vi "DTV&EnQueue.vi"(0 "ModuleAdmin In":refnum<class "ModuleAdmin.lvclass">, 1 "Enqueue Type (Enqueue)":T1=enum."Enqueue", 5 "Message":string, 7 "Message Data":variant, 9 "Class":refnum<class "SensorBase.lvclass">, 11 "Error In":errorcluster, 12 "QueueArrayEntry(QMH)":T2) -> (4 "ModuleAdmin Out":refnum<class "ModuleAdmin.lvclass">, 6 "MessageQueue Out":refnum<queue>, 8 "VariantData":variant, 15 "Error Out":errorcluster)   [LabVIEW 2018, in "SensorPlugins.lvlib"]
doc: "Converts the module data to a variant and places the data in a queue based upon the queue entry and the Enqueue type."
uses:
  SensorPlugins.lvlib
  SensorBaseClass/SensorBase.lvclass
  <userlib>/NIST/ModuleAdminLib/ModuleAdmin/ModuleAdmin.lvclass
  <userlib>/NIST/ModuleAdminLib/ModuleAdmin/TypeDefinitions/QueueEntry.ctl
  <userlib>/NIST/ModuleAdminLib/ModuleAdmin/TypeDefinitions/QueueType.ctl
  clMessage.ctl
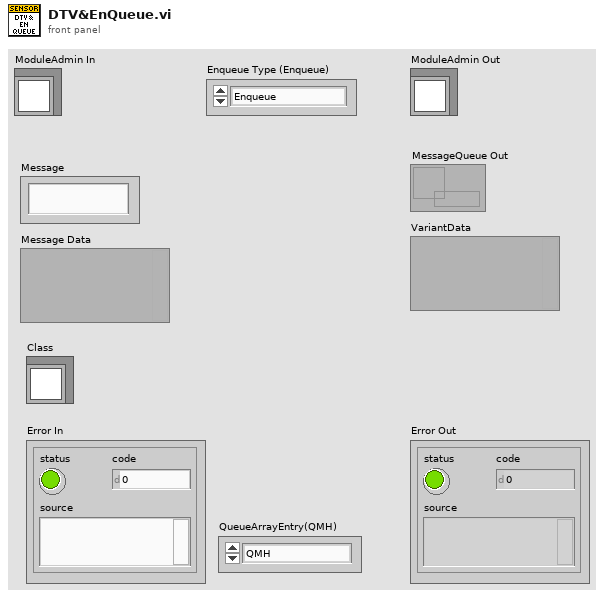
[diagram p1: front panel]
types:
  T1 = typedef "ModuleAdmin.lvlib/ModuleAdmin.lvclass/QueueType.ctl" = enum16{"EnqueueAtFront", "Enqueue", "Lossy Enqueue"}
  T2 = typedef "ModuleAdmin.lvlib/ModuleAdmin.lvclass/QueueEntry.ctl" = enum16{"QMH", "Class Data", "Data Loop", "Queue 4", "Queue 5", "Queue 6", "Queue 7", "Queue 8", "Queue 9", "Queue 10"}
  T3 = typedef "SensorPlugins.lvlib/clMessage.ctl" = cluster{"Message":string, "Message Data":variant, "Class":refnum<class "SensorBase.lvclass">}
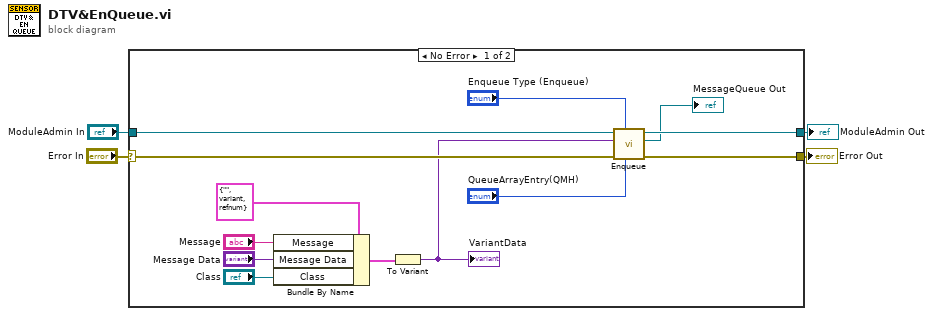
[diagram p0: block diagram]
diagram:
  n1 = case shown="No Error" "Error In" {
    selector: "Error In" -> [w16 w19]
    tunnel: [w8 w19] -> w3
    tunnel: "ModuleAdmin In" -> [w17 w18]
    tunnel: [w7 w18] -> w1
    frame No Error {
      n2 = Bundle By Name(cluster=T3 {"Message"="", "Message Data"=variant, "Class"=refnum} ("clMessage"), "Message"="Message", "Message Data"="Message Data", "Class"="Class") -> (w12:T3)
      n3 = To Variant(anything=w12) -> (Variant=w10:variant)
      "VariantData" <- w10
      n4 = call <userlib>:"Enqueue.vi"("QueueArrayEntry(QMH)"="QueueArrayEntry(QMH)", "Enqueue Type (Enqueue)"="Enqueue Type (Enqueue)", "error in (no error)"=w16, "Queue Element"=w10, "ModuleAdmin In"=w17) -> ("error out"=w8:errorcluster, "MessageQueue Out"=→"MessageQueue Out":refnum<queue>, "ModuleAdmin Out"=w7:refnum<class "ModuleAdmin.lvclass">)  [unwired: 4 in]
    }
    frame Error {
    }
  }
  "Error Out" <- w3
  "ModuleAdmin Out" <- w1
